vi "Acquisition Message Loop.vi"(8 "error in (no error)":errorcluster, 11 "Message Queues":T5) -> (0 "error out":errorcluster)   [LabVIEW 2018, in "Acquisition.lvlib"]
doc: "Message loop for handling messages pertaining to the acquisition of data from the hardware."
uses:
  Acquisition.lvlib
  Support/Message Queue/All Message Queues.ctl
  Support/Message Queue/Message Cluster.ctl
  Controls/Data Queue.ctl
  Controls/Acquired Data.ctl
  Controls/Data Notifier.ctl
  Settings/Settings.ctl
  Hardware Configuration.ctl
  Logging/Logging Configuration.ctl
  <vilib>/addons/database/Connection.llb/Conn ObjectReference.ctl
  Controls/Location Ring.ctl
  Controls/Time Remaining.ctl
  Acquisition State.ctl
  <vilib>/Utility/error.llb/Error Cluster From Error Code.vi
  <vilib>/ErrorRing/Error Ring.xnode
  support/Message Queue/Message Queue.lvlib
  <vilib>/addons/database/NI_Database_API.lvlib
  Logging/Logging.lvlib
  Settings/Settings.lvlib
panel:
  in  "Config & Calibration Data":T1={"Hardware Configuration"={"COM Port"="", "Reference Distance"=0.0, "Sensor SN"=""}, "Logging Configuration"={"Log File Base Path"=path "", "Datafile Ref"=refnum, "Database Ref"=refnum}, "UI Refs"={"Start Ref"=refnum, "Settings Ref"=refnum, "Stop Ref"=refnum, "Exit Ref"=refnum, "Status Ref"=refnum, "Data Ref"=refnum, "StatusBox Ref"=refnum, "Location Ref"=refnum, "Operator Ref"=refnum, "Time Ref"=refnum, "Test in Progess Ref"=refnum}, "Calibration Data"={"calibrationID"=0, "operatorID"=0, "sensorID"=0, "start_time"="", "end_time"="", "offset"=0.0, "offset_units"="", "ring_time"=0.0, "error"=0.0, "Passed"=0, "data_storage_location"="", "comments"=""}, "Time Elapsed"=0, "Samples Required"=480} {"Hardware Configuration"."Reference Distance" format="%.3g"}
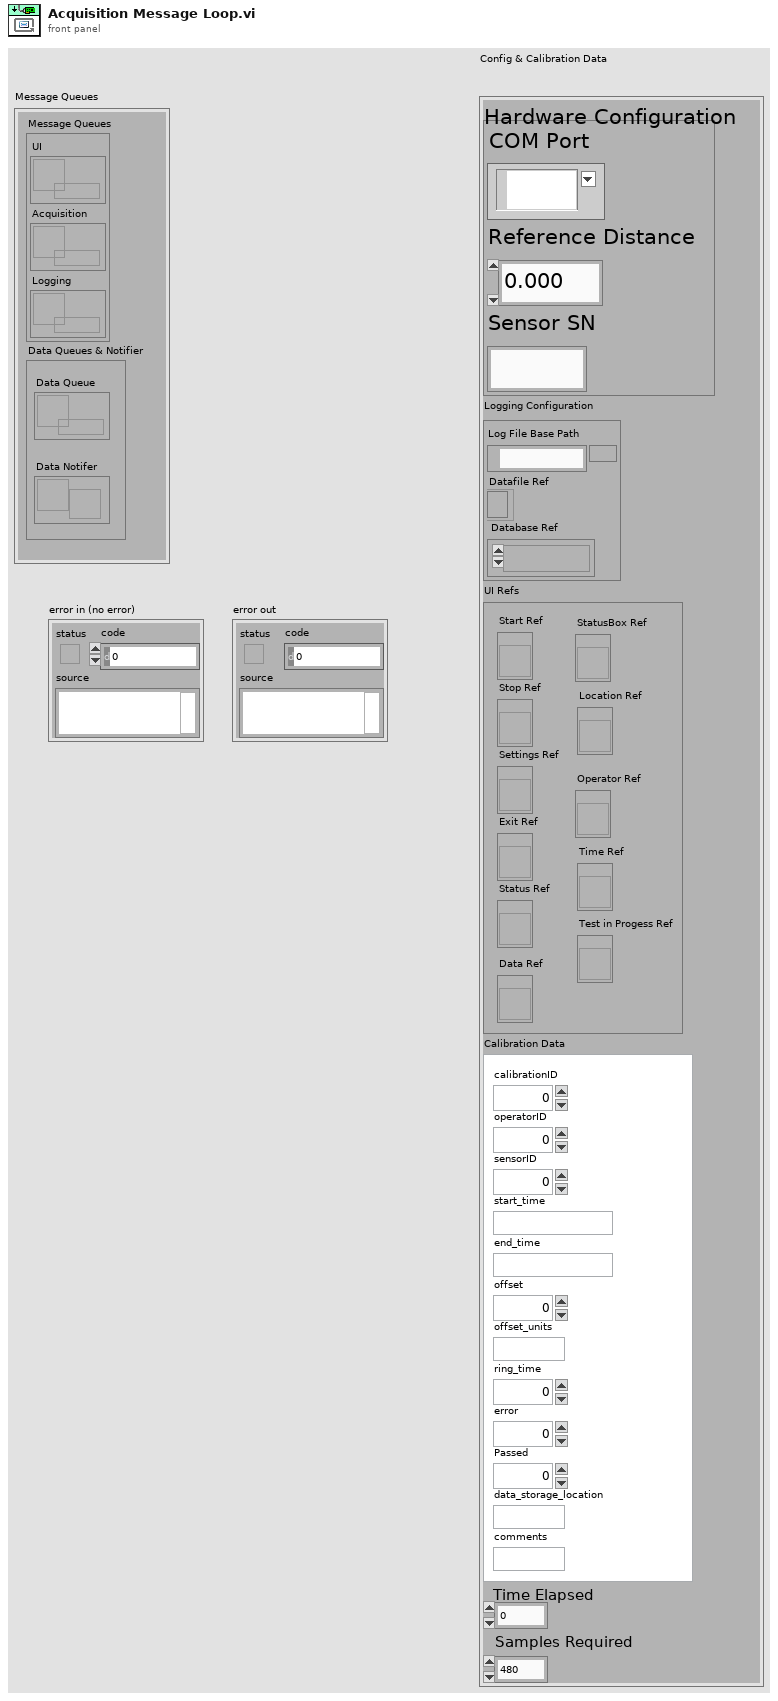
[diagram p1: front panel]
types:
  T1 = typedef "Settings.lvlib/Settings.ctl" = cluster{"Hardware Configuration":T2, "Logging Configuration":T3, "UI Refs":cluster{"Start Ref":refnum<vi>, "Settings Ref":refnum<vi>, "Stop Ref":refnum<vi>, "Exit Ref":refnum<vi>, "Status Ref":refnum<vi>, "Data Ref":refnum<vi>, "StatusBox Ref":refnum<vi>, "Location Ref":refnum<vi>, "Operator Ref":refnum<vi>, "Time Ref":refnum<vi>, "Test in Progess Ref":refnum<vi>}, "Calibration Data":cluster{"calibrationID":u16, "operatorID":u16, "sensorID":u16, "start_time":string, "end_time":string, "offset":dbl, "offset_units":string, "ring_time":dbl, "error":dbl, "Passed":u8, "data_storage_location":string, "comments":string}, "Time Elapsed":u16, "Samples Required":u16}
  T2 = typedef "Acquisition.lvlib/Hardware Configuration.ctl" = cluster{"COM Port":refnum<visa-resource-name>, "Reference Distance":dbl, "Sensor SN":string}
  T3 = typedef "Logging.lvlib/Logging Configuration.ctl" = cluster{"Log File Base Path":path, "Datafile Ref":refnum<file>, "Database Ref":T4}
  T4 = typedef "NI_Database_API.lvlib/Conn ObjectReference.ctl" = refnum<k1>
  T5 = typedef "Message Queue.lvlib/All Message Queues.ctl" = cluster{"Message Queues":cluster{"UI":refnum<queue>, "Acquisition":refnum<queue>, "Logging":refnum<queue>}, "Data Queues & Notifier":cluster{"Data Queue":T6, "Data Notifer":T7}}
  T6 = typedef "Data Queue.ctl" = refnum<queue>
  T7 = typedef "Data Notifier.ctl" = refnum<notifier>
  T8 = typedef "Acquisition.lvlib/Acquisition State.ctl" = enum16{"Idle", "Acquiring"}
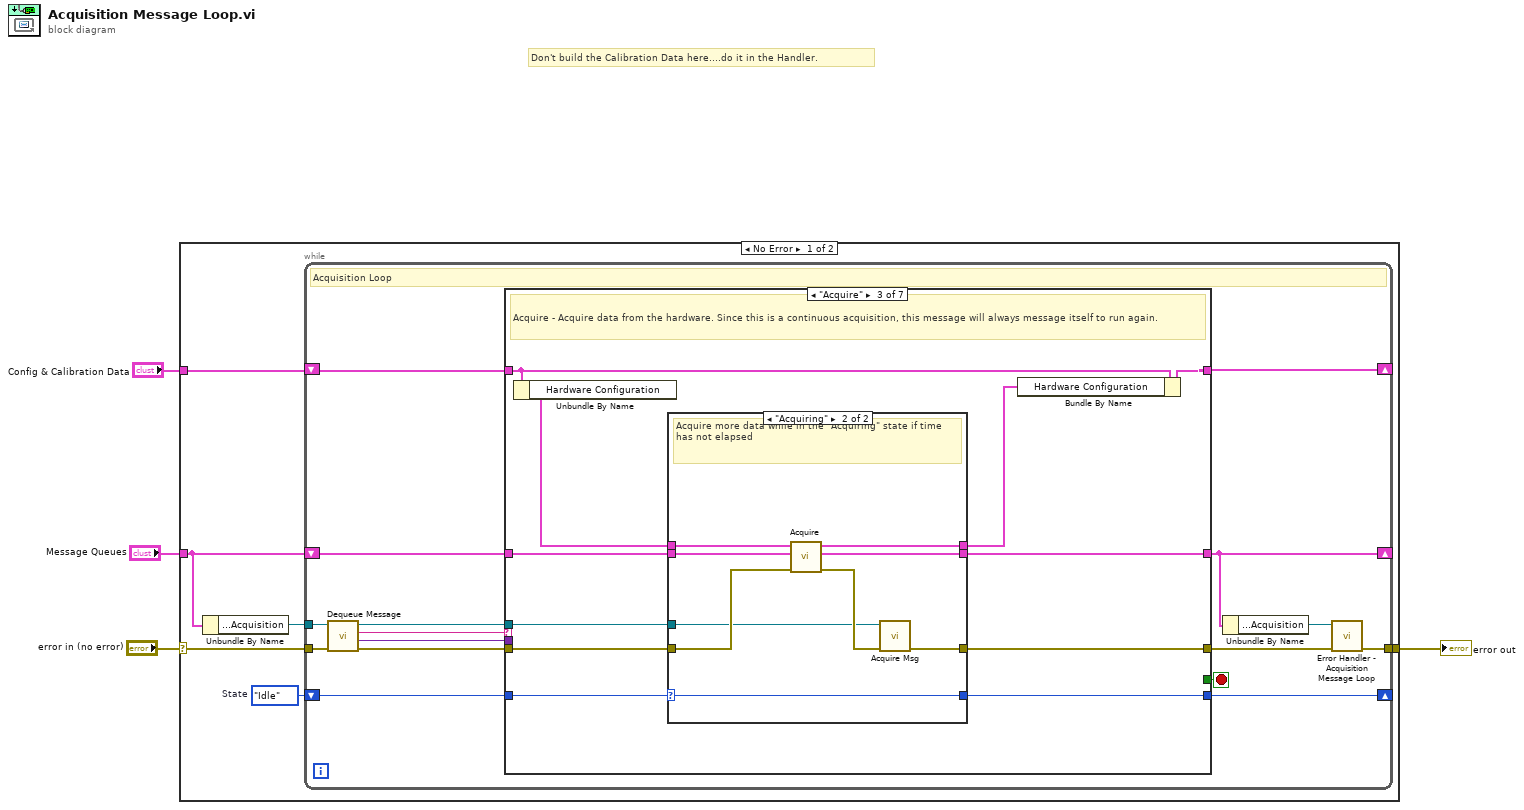
[diagram p0: block diagram]
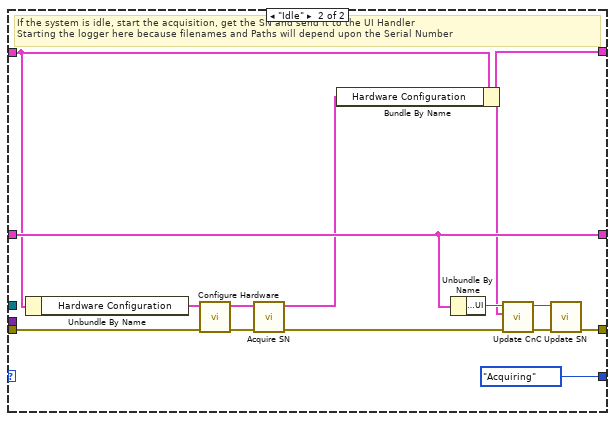
[diagram p4: hidden frame]
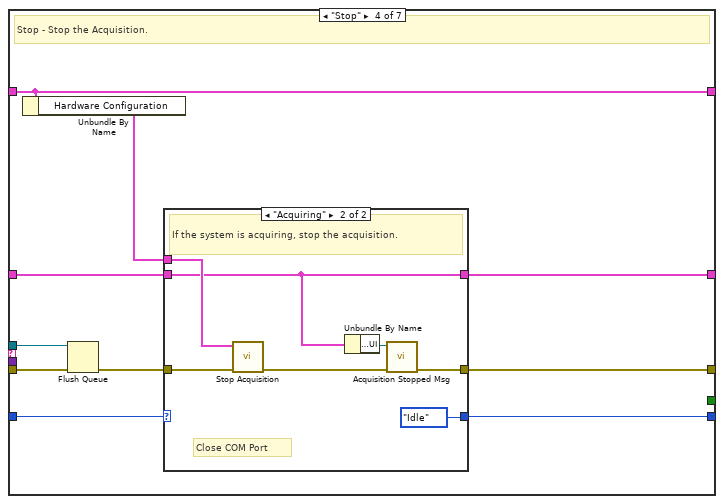
[diagram p6: hidden frame]
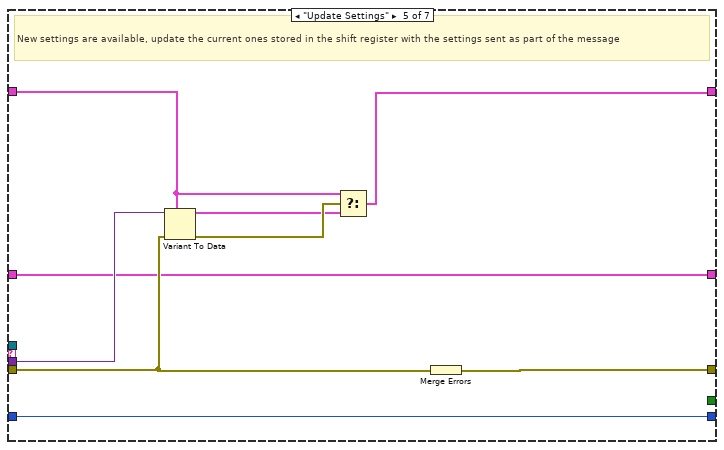
[diagram p8: hidden frame]
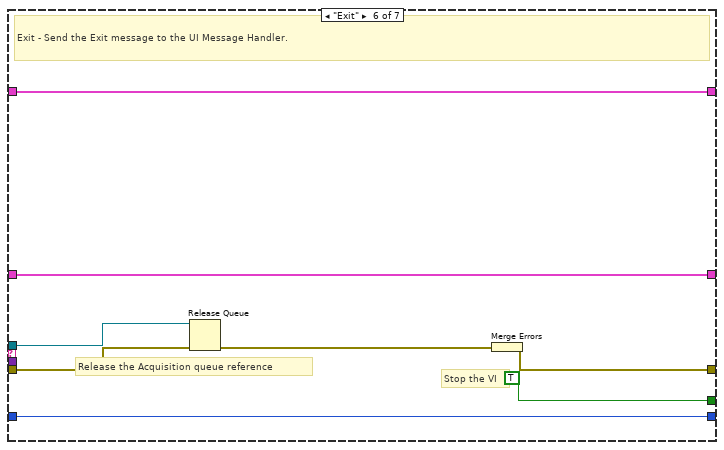
[diagram p9: hidden frame]
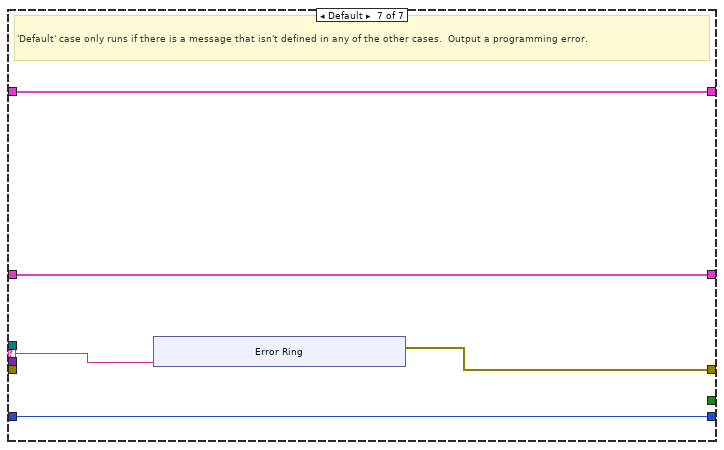
[diagram p10: hidden frame]
diagram:
  # "Don't build the Calibration Data here....do it in the Handler."
  n1 = case shown="No Error" "error in (no error)" {
    selector: "error in (no error)" -> [w8 w132]
    tunnel: "Message Queues" -> [w6 _]
    tunnel: [w9 w132] -> w3
    tunnel: "Config & Calibration Data" -> [w5 _]
    frame No Error {
      w7 = Acquisition_State."Idle"  # State
      n2 = Unbundle By Name(w6) -> ("Message Queues.Acquisition"=w10:refnum<queue>)
      n3 = while {
        tunnel: w10 -> [w21]
        shift-right: [w19] -> _
        shift-left: w7 -> [w20]
        tunnel: w8 -> [w25]
        tunnel: [w18] -> w9
        shift-right: [w14] -> _
        shift-left: w6 -> [w15]
        shift-right: [w12] -> _
        shift-left: w5 -> [w11]
        stop <- w26 stop-if-true
        # "Acquisition Loop"
        n4 = call "Dequeue Message.vi"("error in (no error)"=w25, "Message Queue"=w21) -> ("error out"=w24:errorcluster, "Message Data"=w22:variant, "Message"=w23:string, "dup Message Queue"=w16:refnum<queue>)  [unwired: 6 in]
        n5 = case "Message Cases" shown="\"Acquire\"" w23 {
          selector: w23 -> [_ _ _ _ _ _ w122]
          tunnel: w16 -> [_ w38 w68 w85 _ w115 _]
          tunnel: w24 -> [w30 w39 w67 w87 w108 w117 _]
          tunnel: [w30 w40 w69 w92 w111 w118 w123] -> w17
          tunnel: [_ _ _ _ _ TRUE _] -> w26
          tunnel: w22 -> [_ w33 _ _ w110 _ _]
          tunnel: w20 -> [w29 w36 w65 w91 w107 w114 w124]
          tunnel: [w29 w37 w66 w90 w107 w114 w124] -> w19
          tunnel: w15 -> [w28 w35 w64 w89 w106 w113 w121]
          tunnel: [w28 w34 w63 w88 w106 w113 w121] -> w14
          tunnel: [w27 w31 w60 w84 w105 w112 w120] -> w12
          tunnel: w11 -> [w27 w32 w61 w84 w103 w112 w120]
          frame "Initialize" {
            # "Initialize  - Initialize is currently a no-op.  The hardware initialization takes place in the 'Start' message."
          }
          frame "Start" {
            # "Start - Configure and start the acquisition."
            n6 = case shown="\"Acquiring\"" w36 {
              selector: w36 -> [w43 _]
              tunnel: [w44 w52] -> w40
              tunnel: w39 -> [w44 w54]
              tunnel: w38 -> [_ _]
              tunnel: [w43 Acquisition_State."Acquiring" ("Acquisition State")] -> w37
              tunnel: w35 -> [w42 w55]
              tunnel: [w42 w55] -> w34
              tunnel: w33 -> [_ _]
              tunnel: [w41 w45] -> w31
              tunnel: w32 -> [w41 w51]
              frame "Acquiring" {
                # "The system is already acquiring. Ignore the \"Start\" message."
              }
              frame "Idle" {
                # "If the system is idle, start the acquisition, get the SN and send it to the UI Handler\nStarting the logger here because filenames and Paths will depend upon the Serial Number"
                n7 = Unbundle By Name(w51) -> ("Hardware Configuration"=w53:T2)
                n8 = call "Configure Hardware.vi"("error in (no error)"=w54, "Hardware Resources in"=w53) -> ("error out"=w56:errorcluster, "Hardware Resources out"=w57:T2)  [unwired: 8 in]
                n9 = call "Acquire SN.vi"("error in"=w56, "Hardware Configuration in"=w57) -> ("error out"=w46:errorcluster, "Hardware Configuration out"=w50:T2)  [unwired: 8 in]
                n10 = Bundle By Name(cluster=w51, "Hardware Configuration"=w50) -> (w45:T1)
                n11 = Unbundle By Name(w55) -> ("Message Queues.UI"=w49:refnum<queue>)
                n12 = call "Update CnC.vi"("error in"=w46, "Config & Calibration Data"=w45, "UI Queue in"=w49) -> ("error out"=w47:errorcluster, "UI Queue out"=w48:refnum<queue>)  [unwired: 7 in]
                n13 = call "Update SN.vi"("error in (no error)"=w47, "UI Queue in"=w48) -> ("error out"=w52:errorcluster)  [unwired: 8 in, 1 out]
              }
            }
          }
          frame "Acquire" {
            # "Acquire - Acquire data from the hardware. Since this is a continuous acquisition, this message will always message itself to run again."
            n14 = Unbundle By Name(w61) -> ("Hardware Configuration"=w62:T2)
            n15 = case shown="\"Acquiring\"" w65 {
              selector: w65 -> [w72 w81]
              tunnel: [w73 w77] -> w69
              tunnel: w68 -> [_ w75]
              tunnel: w67 -> [w73 w78]
              tunnel: [w70 w82] -> w59
              tunnel: [w72 w81] -> w66
              tunnel: w64 -> [w71 w80]
              tunnel: [w71 w79] -> w63
              tunnel: w62 -> [w70 w74]
              frame "Idle" {
                # "Ignore \"Acquire\" messages when the acquisition is idle."
              }
              frame "Acquiring" {
                # "Acquire more data while in the \"Acquiring\" state if time has not elapsed"
                n16 = call "Acquire.vi"("error in (no error)"=w78, "Message Queues"=w80, "Hardware Resources in"=w74) -> ("error out"=w76:errorcluster, "Message Queues out"=w79:T5, "Hardware Resources out"=w82:T2)  [unwired: 6 in]
                n17 = call "Acquire Msg.vi"("error in (no error)"=w76, "Queue in"=w75) -> ("error out"=w77:errorcluster)  [unwired: 9 in]
              }
            }
            n18 = Bundle By Name(cluster=w61, "Hardware Configuration"=w59) -> (w60:T1)
          }
          frame "Stop" {
            # "Stop - Stop the Acquisition."
            n19 = Unbundle By Name(w84) -> ("Hardware Configuration"=w83:T2)
            n20 = Flush Queue(queue=w85, error in (no error)=w87) -> (error out=w86:errorcluster)  [unwired: 2 out]
            n21 = case shown="\"Acquiring\"" w91 {
              selector: w91 -> [w94 _]
              tunnel: w86 -> [w95 w102]
              tunnel: [w95 w98] -> w92
              tunnel: w83 -> [_ w100]
              tunnel: [w94 Acquisition_State."Idle" ("State")] -> w90
              tunnel: w89 -> [w93 w96]
              tunnel: [w93 w96] -> w88
              frame "Idle" {
                # "The system is already idle. Ignore the \"Stop\" message."
              }
              frame "Acquiring" {
                # "Close COM Port"
                # "If the system is acquiring, stop the acquisition."
                n22 = call "Stop Acquisition.vi"("error in (no error)"=w102, "Hardware Resources in"=w100) -> ("error out"=w101:errorcluster)  [unwired: 9 in]
                n23 = Unbundle By Name(w96) -> ("Message Queues.UI"=w97:refnum<queue>)
                n24 = call "Acquisition Stopped Msg.vi"("error in (no error)"=w101, "Queue in"=w97) -> ("error out"=w98:errorcluster)  [unwired: 9 in]
              }
            }
          }
          frame "Update Settings" {
            # "New settings are available, update the current ones stored in the shift register with the settings sent as part of the message"
            n25 = Variant To Data(error in=w108, type=w103, Variant=w110) -> (data=w104:T1, error out=w109:errorcluster)
            n26 = Select(t=w103, s=w109, f=w104) -> (s? t:f=w105:T1)
            n27 = Merge Errors(w108) -> (w111:errorcluster)
          }
          frame "Exit" {
            # "Release the Acquisition queue reference"
            # "Stop the VI"
            # "Exit - Send the Exit message to the UI Message Handler."
            n28 = Release Queue(queue=w115, error in (no error)=w117) -> (error out=w116:errorcluster)  [unwired: 1 in, 2 out]
            n29 = Merge Errors(w116) -> (w118:errorcluster)
          }
          frame Default {
            # "'Default' case only runs if there is a message that isn't defined in any of the other cases.  Output a programming error."
            n30 = xnode "Error Ring"("parameter 0"=w122) -> ("error out"=w123:errorcluster)
          }
        }
        n31 = Unbundle By Name(w14) -> ("Message Queues.Acquisition"=w13:refnum<queue>)
        n32 = call "Error Handler - Acquisition Message Loop.vi"("error in (no error)"=w17, "Message Queue"=w13) -> ("dup error in"=w18:errorcluster)  [unwired: 8 in, 1 out]
      }
    }
    frame Error {
    }
  }
  "error out" <- w3
